vi "MarkTested.vi"(7 "Enum":enum16{"MarkTested", "MarkNotTested"}(ring), 8 "error in (no error)":errorcluster, 11 "LotData in":refnum<class "LotData.lvclass">) -> (0 "error out":errorcluster, 2 "Message":string, 3 "LotData out":refnum<class "LotData.lvclass">)   [LabVIEW 2012, in "LotData.lvclass"]
uses:
  LotData.lvclass
  <vilib>/addons/database/Auxilliary.llb/DB Tools Parameter Info.ctl
  <vilib>/addons/database/Auxilliary.llb/DB Tools DataTypes.ctl
  <vilib>/addons/database/Auxilliary.llb/DB Tools Parameter Dir.ctl
  LotData.lvclass/LotData.ctl
  <vilib>/addons/database/Connection.llb/DB Tools Open Connec (Path).vi
  <vilib>/addons/database/Command.llb/Cmd Set Parameter Value (C).vi
  <vilib>/addons/database/Command.llb/Cmd Execute.vi
  <vilib>/addons/database/Recordset.llb/Rec Destroy - Command.vi
  <vilib>/addons/database/Command.llb/Cmd Delete.vi
  <vilib>/addons/database/NI_Database_API.lvlib
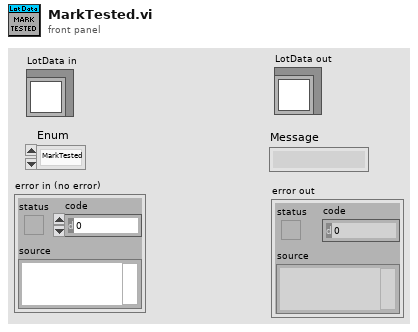
[diagram p1: front panel]
types:
  T1 = typedef "NI_Database_API.lvlib/DB Tools Parameter Info.ctl" = cluster{"parameter name":string, "type":T2, "direction":T3, "value":variant}
  T2 = typedef "NI_Database_API.lvlib/DB Tools DataTypes.ctl" = enum16{"String", "Long (I32)", "Single (SGL)", "Double (DBL)", "Date/Time", "Binary"}
  T3 = typedef "NI_Database_API.lvlib/DB Tools Parameter Dir.ctl" = enum32{"Input", "Output", "Input/Output", "Return Value"}
  T4 = typedef "NI_Database_API.lvlib/Conn ObjectReference.ctl" = refnum<k1>
  T5 = typedef "NI_Database_API.lvlib/Cmd ObjectReference.ctl" = refnum<k1>
  T6 = typedef "NI_Database_API.lvlib/Cmd-Rec Object Reference.ctl" = refnum<k1>
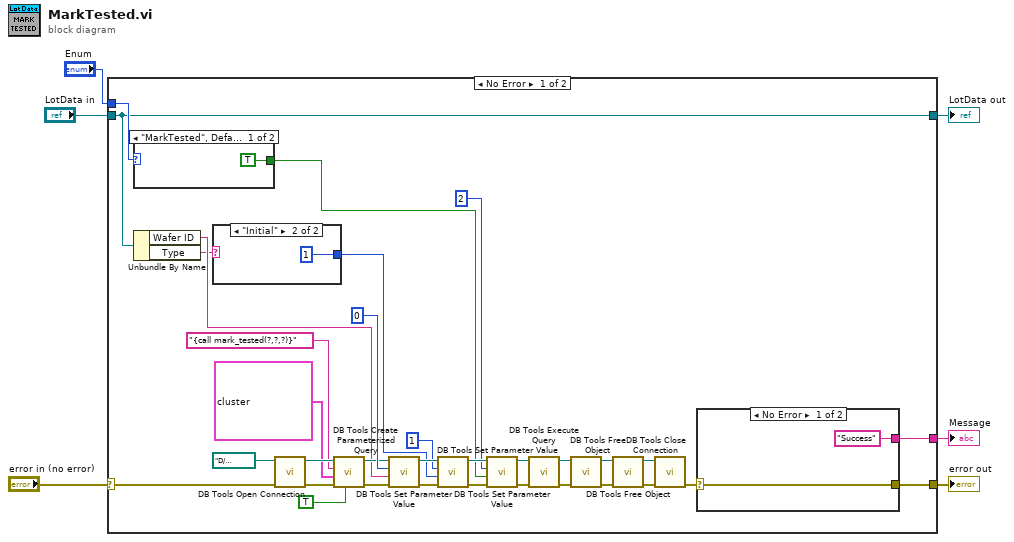
[diagram p0: block diagram]
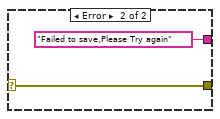
[diagram p2: hidden frame]
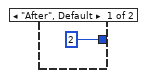
[diagram p3: hidden frame]
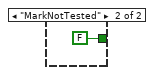
[diagram p4: hidden frame]
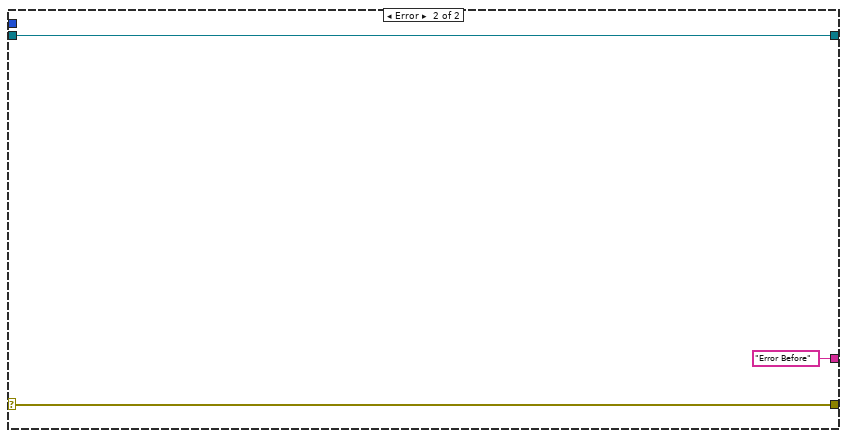
[diagram p5: hidden frame]
diagram:
  n1 = case shown="No Error" "error in (no error)" {
    selector: "error in (no error)" -> [w14 w50]
    tunnel: [w7 w50] -> w5
    tunnel: [w38 w48] -> w3
    tunnel: "LotData in" -> [w38 w48]
    tunnel: "Enum" -> [w39 _]
    tunnel: [w8 "Error Before"] -> w1
    frame No Error {
      n2 = case shown="\"MarkTested\", Default" w39 {
        tunnel: [TRUE ("isTested") FALSE ("isTested")] -> w12
        frame "MarkTested", Default {
        }
        frame "MarkNotTested" {
        }
      }
      n3 = Unbundle By Name(w38) -> ("Wafer ID"=w13:string, "Type"=w11:string)
      n4 = case shown="\"Initial\"" w11 {
        tunnel: [2 1] -> w10
        frame "After", Default {
        }
        frame "Initial" {
        }
      }
      n5 = call-poly <vilib>:"DB Tools Open Connection.vi"("error in (no error)"=w14, "connection information"=path "D:/Program Files (x86)/National Instruments/LabVIEW 2012/Database/epiDataLink.udl") -> ("error out"=w34:errorcluster, "connection reference"=w35:T4)  [unwired: 6 in]
      n6 = call <vilib>:"DB Tools Create Parameterized Query.vi"("stored procedure? (F)"=TRUE, "error in (no error)"=w34, "parameters"=T1[] [{"parameter name"="wafer", "type"=enum."String", "direction"=enum."Input", "value"=variant}, {"parameter name"="test", "type"=enum."Single (SGL)", "direction"=enum."Input", "value"=variant}, {"parameter name"="isTested", "type"=enum."Binary", "direction"=enum."Input", "value"=variant}], "SQL query"="{call mark_tested(?,?,?)}", "connection reference"=w35) -> ("error out"=w31:errorcluster, "command reference"=w30:T5)  [unwired: 2 in, 1 out]
      n7 = call-poly <vilib>:"DB Tools Set Parameter Value.vi"("error in (no error)"=w31, "value"=w13, "parameter index"=0, "command reference"=w30) -> ("error out"=w23:errorcluster, "command reference out"=w22:T5)  [unwired: 4 in]
      n8 = call-poly <vilib>:"DB Tools Set Parameter Value.vi"("error in (no error)"=w23, "value"=w10, "parameter index"=1, "command reference"=w22) -> ("error out"=w20:errorcluster, "command reference out"=w21:T5)  [unwired: 4 in]
      n9 = call-poly <vilib>:"DB Tools Set Parameter Value.vi"("error in (no error)"=w20, "value"=w12, "parameter index"=2, "command reference"=w21) -> ("error out"=w15:errorcluster, "command reference out"=w16:T5)  [unwired: 4 in]
      n10 = call-poly <vilib>:"DB Tools Execute Query.vi"("error in (no error)"=w15, "command reference"=w16) -> ("error out"=w27:errorcluster, "command-recordset reference"=w28:T6)  [unwired: 6 in]
      n11 = call-poly <vilib>:"DB Tools Free Object.vi"("error in (no error)"=w27, "command-recordset reference"=w28) -> ("error out"=w29:errorcluster, "command reference"=w24:T5)  [unwired: 8 in]
      n12 = call-poly <vilib>:"DB Tools Free Object.vi"("error in (no error)"=w29, "command reference"=w24) -> ("error out"=w25:errorcluster, "connection reference"=w26:T4)  [unwired: 8 in]
      n13 = call <vilib>:"DB Tools Close Connection.vi"("error in (no error)"=w25, "connection reference"=w26) -> ("error out"=w9:errorcluster)  [unwired: 5 in]
      n14 = case shown="No Error" w9 {
        selector: w9 -> [w40 w43]
        tunnel: ["Success" "Failed to save,Please Try again"] -> w8
        tunnel: [w40 w43] -> w7
        frame No Error {
        }
        frame Error {
        }
      }
    }
    frame Error {
    }
  }
  "error out" <- w5
  "LotData out" <- w3
  "Message" <- w1
